vi "Merge.vi"(8 "Sort VI":T1, 10 "B":refnum<data-value>[](array[refnum]), 11 "A":refnum<data-value>[](array[refnum])) -> (3 "Merged":refnum<data-value>[](array[refnum]))   [LabVIEW 2020, in "OOPanel.lvlib" / "ArrayManager.lvclass"]
uses:
  <vilib>/IlluminatedG/IG OOPanel/OOPanel/ArrayManager/ArrayManager.lvclass
  <vilib>/IlluminatedG/IG OOPanel/OOPanel/ArrayManager/ArrayManager.lvclass/ArrayManager.ctl
  <vilib>/IlluminatedG/IG OOPanel/OOPanel/ArrayPanel/ArrayPanel.lvclass
  C:/dev/IlluminatedG/.lv-oopanel/OOPanel/Panel/Panel.lvclass
  <vilib>/IlluminatedG/IG OOPanel/OOPanel/ArrayManager/Sort VI Type.ctl
  <vilib>/IlluminatedG/IG OOPanel/OOPanel/Panel/Panel.lvclass
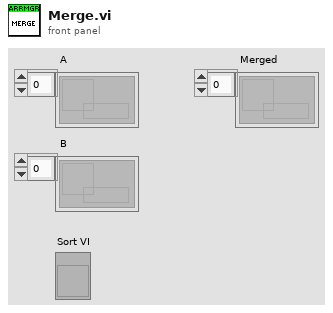
[diagram p1: front panel]
types:
  T1 = typedef "OOPanel.lvlib/ArrayManager.lvclass/Sort VI Type.ctl" = refnum<vi>
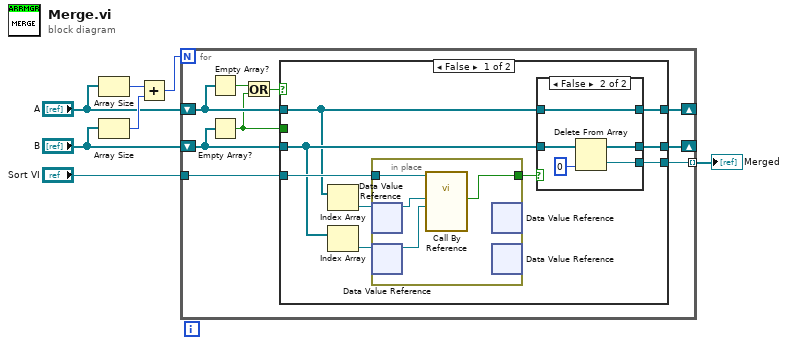
[diagram p0: block diagram]
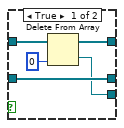
[diagram p2: hidden frame]
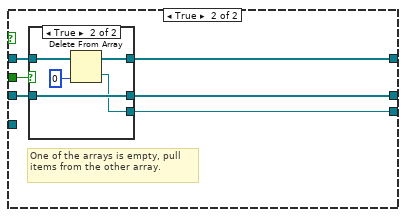
[diagram p3: hidden frame]
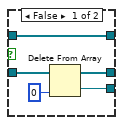
[diagram p4: hidden frame]
diagram:
  n1 = Array Size(array="A") -> (size(s)=w7:i32)
  n2 = Array Size(array="B") -> (size(s)=w6:i32)
  n3 = Add(x=w7, y=w6) -> (x+y=w5:i32)
  n4 = for {
    N: w5 -> [_]
    shift-right: [w15] -> _
    shift-left: "A" -> [w12]
    shift-right: [w14] -> _
    shift-left: "B" -> [w11]
    tunnel: "Sort VI" -> [w16]
    tunnel: [w13] -> w1 mode=indexing
    n5 = Empty Array?(array=w12) -> (empty?=w10:bool)
    n6 = Empty Array?(array=w11) -> (empty?=w8:bool)
    n7 = Or(x=w10, y=w8) -> (x .or. y?=w9:bool)
    n8 = case shown="False" w9 {
      tunnel: w16 -> [w23 _]
      tunnel: [w21 w40] -> w15
      tunnel: [w20 w42] -> w14
      tunnel: [w19 w41] -> w13
      tunnel: w12 -> [w17 w44]
      tunnel: w11 -> [w18 w43]
      tunnel: w8 -> [_ w45]
      frame False {
        n9 = Index Array(array=w17) -> (element=w25:refnum<data-value>)  [unwired: 1 in]
        n10 = Index Array(array=w18) -> (element=w24:refnum<data-value>)  [unwired: 1 in]
        n11 = in-place {
          in-place-border: w23 -> [w39]
          in-place-border: [w36] -> w22
          n12 = in-place-dvr #1(w25) -> (w38:refnum<class "ArrayPanel.lvclass">)  [unwired: 1 out]
          n13 = in-place-dvr #2(w24) -> (w37:refnum<class "ArrayPanel.lvclass">)  [unwired: 1 out]
          n14 = call-by-ref "?"(reference=w39, "Panel B"=w37, "Panel A"=w38) -> ("A < B"=w36:bool)  [unwired: 10 in, 2 out]
          n15 = in-place-dvr #1() -> ()  [unwired: 1 in, 2 out]
          n16 = in-place-dvr #2() -> ()  [unwired: 1 in, 2 out]
        }
        n17 = case shown="False" w22 {
          tunnel: w18 -> [w27 w34]
          tunnel: w17 -> [w30 w32]
          tunnel: [w28 w32] -> w21
          tunnel: [w27 w33] -> w20
          tunnel: [w26 w31] -> w19
          frame True {
            n18 = Delete From Array(array=w30, index=0) -> (deleted portion=w26:refnum<data-value>, array with subset deleted=w28:refnum<data-value>[])  [unwired: 1 in]
          }
          frame False {
            n19 = Delete From Array(array=w34, index=0) -> (deleted portion=w31:refnum<data-value>, array with subset deleted=w33:refnum<data-value>[])  [unwired: 1 in]
          }
        }
      }
      frame True {
        # "One of the arrays is empty, pull items from the other array."
        n20 = case shown="True" w45 {
          tunnel: w44 -> [w47 w54]
          tunnel: w43 -> [w50 w55]
          tunnel: [w49 w55] -> w42
          tunnel: [w48 w53] -> w41
          tunnel: [w47 w51] -> w40
          frame False {
            n21 = Delete From Array(array=w50, index=0) -> (deleted portion=w48:refnum<data-value>, array with subset deleted=w49:refnum<data-value>[])  [unwired: 1 in]
          }
          frame True {
            n22 = Delete From Array(array=w54, index=0) -> (deleted portion=w53:refnum<data-value>, array with subset deleted=w51:refnum<data-value>[])  [unwired: 1 in]
          }
        }
      }
    }
  }
  "Merged" <- w1
